vi "Connection Dropped.vi"(8 "error in (no error)":errorcluster, 11 "WS Test Client Subscriber in":refnum<class "WS Test Client Subscriber.lvclass">) -> (0 "error out":errorcluster, 3 "WS Test Client Subscriber out":refnum<class "WS Test Client Subscriber.lvclass">)   [LabVIEW 2021, in "Echo Broadcast Test With Server Manager.lvlib" / "WS Test Client Subscriber.lvclass"]
uses:
  WS Test Client Subscriber.lvclass
  C:/Program Files/National Instruments/LabVIEW 2021/vi.lib/ActorFramework/Actor/Actor.lvclass
  <vilib>/ActorFramework/Actor/Actor.lvclass/Actor.ctl
  <vilib>/ActorFramework/Message Enqueuer/Message Enqueuer.lvclass/Message Enqueuer.ctl
  <vilib>/ActorFramework/Message Enqueuer/Init from Existing Queue.vi
  <vilib>/ActorFramework/Message Enqueuer/Enqueue.vi
  <vilib>/ActorFramework/Stop Msg/Stop Msg.lvclass
  C:/Program Files/National Instruments/LabVIEW 2021/vi.lib/ActorFramework/Message/Message.lvclass
  <vilib>/Utility/LVClass/Get LV Class Name.vi
  <resource>/AFDebug/Generate Trace for Message.vi
  <vilib>/ActorFramework/Message Priority Queue/Priority Enqueue.vi
  <vilib>/ActorFramework/Message Enqueuer/Message Enqueuer.lvclass
  WS Test Client Subscriber.lvclass/WS Test Client Subscriber.ctl
  <vilib>/ActorFramework/Actor/Actor.lvclass
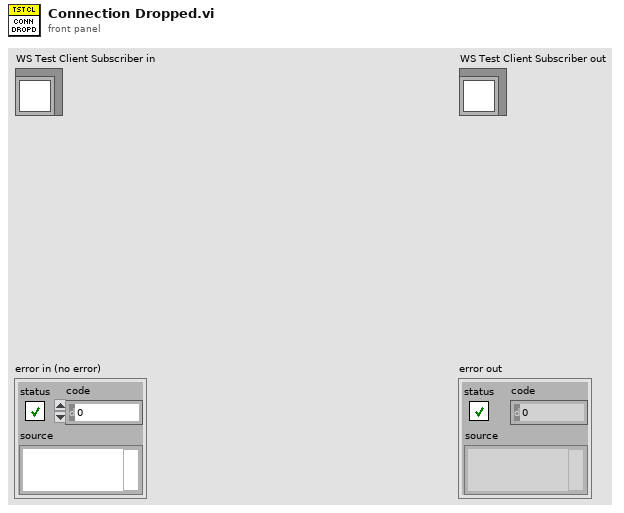
[diagram p1: front panel]
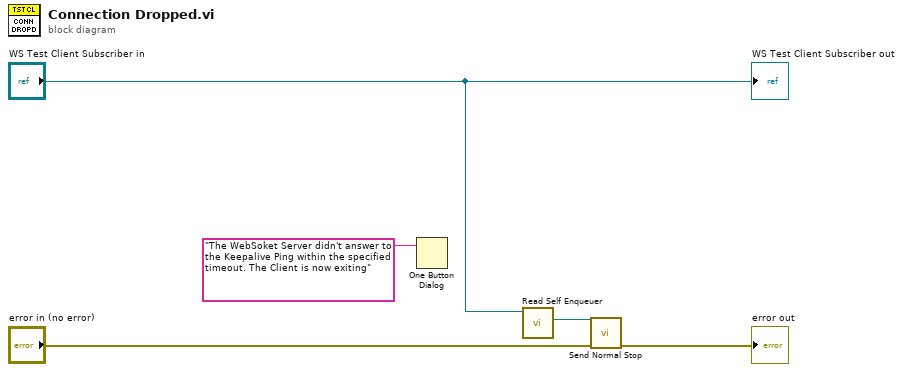
[diagram p0: block diagram]
diagram:
  n1 = One Button Dialog(message="The WebSoket Server didn't answer to the Keepalive Ping within the specified timeout. The Client is now exiting") -> ()  [unwired: 1 in, 1 out]
  n2 = call <vilib>:"Read Self Enqueuer.vi"("Actor"="WS Test Client Subscriber in") -> ("Self Enqueuer"=w1:refnum<class "Message Enqueuer.lvclass">)  [unwired: 10 in]
  n3 = call <vilib>:"Send Normal Stop.vi"("error in (no error)"="error in (no error)", "Message Enqueuer"=w1) -> ("error out"=→"error out":errorcluster)  [unwired: 9 in]
  "WS Test Client Subscriber out" <- "WS Test Client Subscriber in"
